vi "FGEN-WFMs.vi"() -> ()   [LabVIEW 2018]
uses:
  <vilib>/measure/NI_MABase.lvlib
panel:
  in  "Np":i32
  in  "Ns":i32
  in  "fs (input)":dbl
  out "Ns (FGen)":dbl=1000.0
  out "fs (FGEN)":dbl=1000.0
  in  "fp (wfm)":dbl=10000.0 format="%.10f"
  out "Perturbation Waveform":waveform(dbl)(graph)
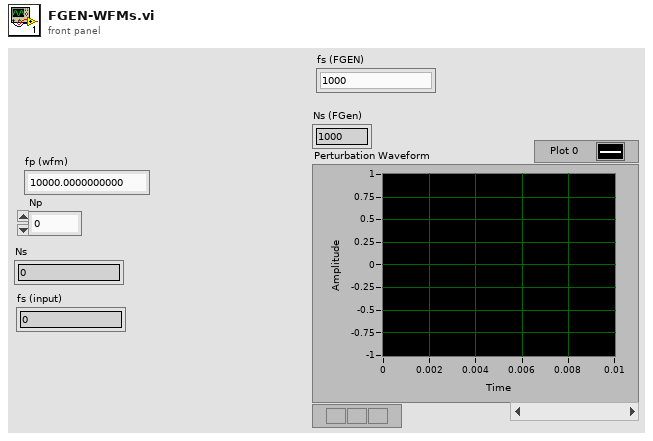
[diagram p1: front panel]
types:
  T1 = enum16{"Sine Wave", "Triangle Wave", "Square Wave", "Sawtooth Wave"}
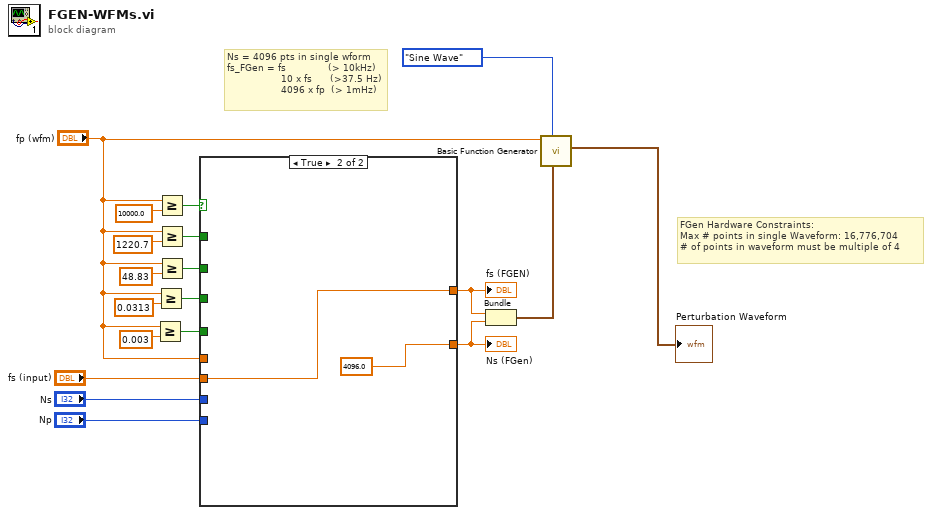
[diagram p0: block diagram]
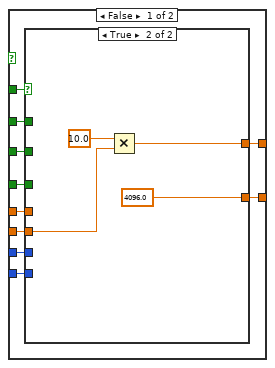
[diagram p2: hidden frame]
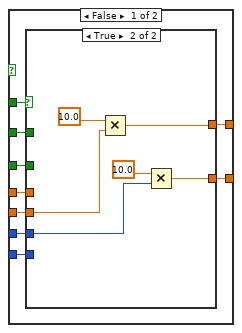
[diagram p3: hidden frame]
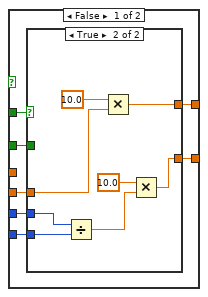
[diagram p4: hidden frame]
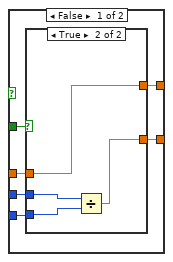
[diagram p5: hidden frame]
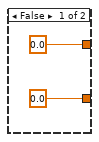
[diagram p6: hidden frame]
diagram:
  # "Ns = 4096 pts in single wform\nfs_FGen = fs              (> 10kHz)\n                  10 x fs      (>37.5 Hz)\n                  4096 x fp  (> 1mHz)"
  # "FGen Hardware Constraints:\nMax # points in single Waveform: 16,776,704\n# of points in waveform must be multiple of 4"
  n1 = Greater Or Equal?(x="fp (wfm)", y=0.003) -> (x >= y?=w2:bool)
  n2 = Greater Or Equal?(x="fp (wfm)", y=0.0313) -> (x >= y?=w3:bool)
  n3 = Greater Or Equal?(x="fp (wfm)", y=10000.0) -> (x >= y?=w15:bool)
  n4 = Greater Or Equal?(x="fp (wfm)", y=1220.7) -> (x >= y?=w8:bool)
  n5 = Greater Or Equal?(x="fp (wfm)", y=48.83) -> (x >= y?=w16:bool)
  n6 = case shown="True" w15 {
    tunnel: [w27 w76] -> w12
    tunnel: [w28 4096.0 ("Fs")] -> w11
    tunnel: w16 -> [w29 _]
    tunnel: "fs (input)" -> [w26 w76]
    tunnel: w8 -> [w25 _]
    tunnel: "fp (wfm)" -> [w24 _]
    tunnel: "Ns" -> [w23 _]
    tunnel: w3 -> [w22 _]
    tunnel: w2 -> [w21 _]
    tunnel: "Np" -> [w20 _]
    frame False {
      n7 = case shown="True" w25 {
        tunnel: w29 -> [w37 _]
        tunnel: [w35 4096.0 ("Fs")] -> w28
        tunnel: [w36 w72] -> w27
        tunnel: w26 -> [w38 w74]
        tunnel: w24 -> [w34 _]
        tunnel: w23 -> [w33 _]
        tunnel: w22 -> [w32 _]
        tunnel: w21 -> [w31 _]
        tunnel: w20 -> [w30 _]
        frame False {
          n8 = case shown="True" w37 {
            tunnel: [w42 w70] -> w36
            tunnel: [w41 w66] -> w35
            tunnel: w38 -> [w43 w69]
            tunnel: w34 -> [_ _]
            tunnel: w33 -> [w40 w67]
            tunnel: w32 -> [w45 _]
            tunnel: w31 -> [w44 _]
            tunnel: w30 -> [w39 _]
            frame False {
              n9 = case shown="True" w45 {
                tunnel: w44 -> [w51 _]
                tunnel: w43 -> [w48 w64]
                tunnel: [w50 w63] -> w42
                tunnel: [w49 w58] -> w41
                tunnel: w40 -> [w47 w62]
                tunnel: w39 -> [w46 w61]
                frame False {
                  n10 = case shown="True" w51 {
                    tunnel: [0.0 ("y") w57] -> w50
                    tunnel: [0.0 ("y") w54] -> w49
                    tunnel: w48 -> [_ w57]
                    tunnel: w47 -> [_ w56]
                    tunnel: w46 -> [_ w55]
                    frame False {
                    }
                    frame True {
                      n11 = Divide(x=w56, y=w55) -> (x/y=w54:dbl)
                    }
                  }
                }
                frame True {
                  n12 = Divide(x=w62, y=w61) -> (x/y=w59:dbl)
                  n13 = Multiply(x=10.0, y=w64) -> (x*y=w63:dbl)
                  n14 = Multiply(x=10.0, y=w59) -> (x*y=w58:dbl)
                }
              }
            }
            frame True {
              n15 = Multiply(x=10.0, y=w69) -> (x*y=w70:dbl)
              n16 = Multiply(x=10.0, y=w67) -> (x*y=w66:dbl)
            }
          }
        }
        frame True {
          n17 = Multiply(x=10.0, y=w74) -> (x*y=w72:dbl)
        }
      }
    }
    frame True {
    }
  }
  "fs (FGEN)" <- w12
  "Ns (FGen)" <- w11
  n18 = Bundle("fs (input)"=w12, "Fs"=w11) -> (w17:cluster{"fs (input)":dbl, "Fs":dbl})  [unwired: 1 in]
  n19 = call <vilib>:"Basic Function Generator.vi"("sampling info"=w17, "signal type"=T1."Sine Wave" ("Signal Type"), "frequency"="fp (wfm)") -> ("signal out"=→"Perturbation Waveform":waveform(dbl))  [unwired: 6 in, 2 out]
